vi "Voice coil response and camera trigger_latest.vi"() -> ()   [LabVIEW 2020]
uses:
  <vilib>/DAQmx/read.llb/DAQmx Read (Analog Wfm 1Chan NSamp).vi
  <vilib>/DAQmx/write.llb/DAQmx Write (Analog 1D Wfm NChan NSamp).vi
  <vilib>/DAQmx/create/channels.llb/DAQmx Create Channel (AO-Voltage-Basic).vi
  <vilib>/DAQmx/configure/timing.llb/DAQmx Timing (Use Waveform).vi
  <vilib>/DAQmx/create/channels.llb/DAQmx Create Channel (AI-Voltage-Basic).vi
  <vilib>/DAQmx/configure/timing.llb/DAQmx Timing (Sample Clock).vi
  <vilib>/DAQmx/miscellaneous.llb/DAQmx Fill In Error Info.vi
  <vilib>/Analysis/polynomials.llb/Subtract Polynomials (DBL).vi
  <vilib>/measure/NI_MABase.lvlib
  <vilib>/Analysis/NI_AALPro.lvlib
panel:
  in  "Stop 3":bool
  out "fractional index or x":dbl=9999.0
  out "x/y":dbl=0.5800133152535774
  out "Modified sawtooth input(red) and original sawtooth input (blue)":waveform(dbl)[](graph)=[{"t0"=timestamp(0 s since 1904-01-01), "dt"=0.0001, "Y"=array[10000 elements]}, {"t0"=timestamp(0 s since 1904-01-01), "dt"=0.0001, "Y"=array[10000 elements]}]
  out "intercept":dbl=-0.029693873912173534
  out "slope":dbl=1.09
  out "Linear fit (red), Voice coil response (blue) and Subtracted fit from voice coil response (green)":waveform(dbl)[](graph)=[{"t0"=timestamp(3778592903.950374 s since 1904-01-01), "dt"=9.999999999999999e-05, "Y"=array[10000 elements], "attributes"=variant("NI_ChannelName"=variant(string "Dev1/ai6"), "NI_UnitDescription"=variant(string "Volts"))}, {"t0"=timestamp(0 s since 1904-01-01), "dt"=0.0001, "Y"=array[10000 elements]}, {"t0"=timestamp(0 s since 1904-01-01), "dt"=0.0001, "Y"=array[10000 elements]}]
  in  "Stop 2":bool
  out "Sample Rate":dbl format="%0.2f"
  in  "Camera trigger delay (degrees)":dbl=180.0
  in  "Exposure time (ms)":dbl=1000.0
  in  "Sawtooth Offset":dbl
  in  "Sawtooth Amplitude":dbl=0.2
  in  "Sawtooth Phase":dbl=170.0
  out "Sawtooth input (blue), Voice coil response (red), Voice coil response - Sawtooth input (green)":waveform(dbl)[](graph)=[{"t0"=timestamp(0 s since 1904-01-01), "dt"=0.0001, "Y"=array[10000 elements]}, {"t0"=timestamp(3778592903.950374 s since 1904-01-01), "dt"=9.999999999999999e-05, "Y"=array[10000 elements], "attributes"=variant("NI_ChannelName"=variant(string "Dev1/ai6"), "NI_UnitDescription"=variant(string "Volts"))}, {"t0"=timestamp(0 s since 1904-01-01), "dt"=0.0001, "Y"=array[10000 elements]}]
  out "LabVIEW generated Sawtooth input (blue) and Camera trigger (red)":waveform(dbl)[](graph)=[{"t0"=timestamp(0 s since 1904-01-01), "dt"=0.0001, "Y"=array[10000 elements]}, {"t0"=timestamp(0 s since 1904-01-01), "dt"=0.0001, "Y"=array[10000 elements]}]
  # "Synchronization Settings"
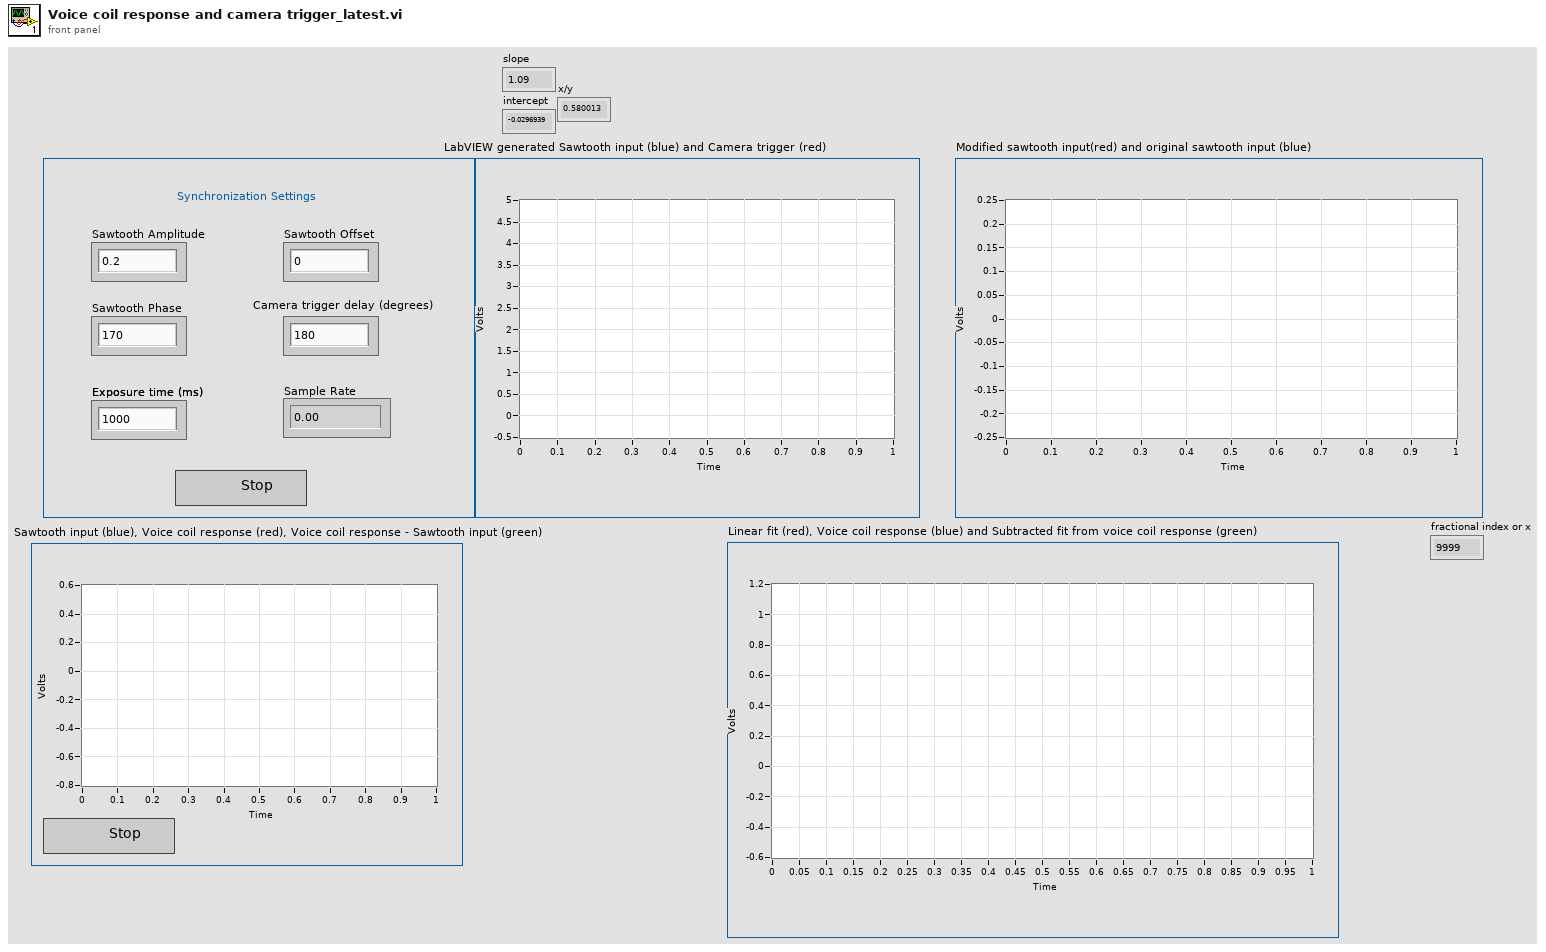
[diagram p1: front panel]
types:
  T1 = cluster{"slope min":dbl, "slope max":dbl, "intercept min":dbl, "intercept max":dbl}
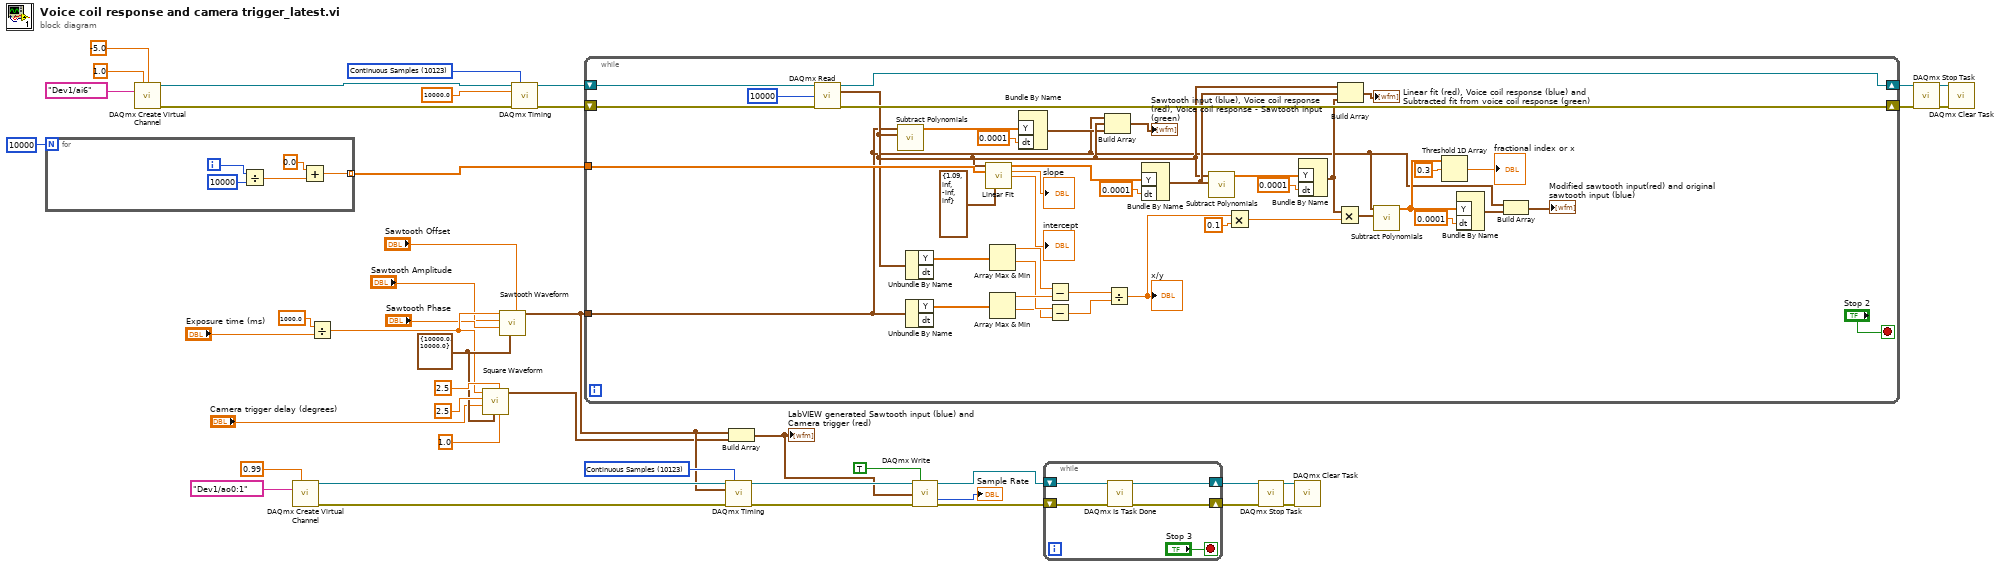
[diagram p0: block diagram]
diagram:
  w31 = 10123 items=["Finite Samples"=10178, "Continuous Samples"=10123, "Hardware Timed Single Point"=12522] ("sample mode")
  w36 = cluster{"Fs":dbl, "#s":dbl} {"Fs"=10000.0, "#s"=10000.0} ("sampling info")
  w41 = 10123 items=["Finite Samples"=10178, "Continuous Samples"=10123, "Hardware Timed Single Point"=12522] ("sample mode")
  n1 = for {
    N: 10000 -> [_]
    tunnel: [w45] -> w16 mode=indexing
    i -> [w49]
    n2 = Divide(x=w49, y=10000) -> (x/y=w46:dbl)
    n3 = Add(x=0.0, y=w46) -> (x+y=w45:dbl)
  }
  n4 = call-poly <vilib>:"DAQmx Create Virtual Channel.vi"("maximum value"=1.0, "minimum value"=-5.0, "physical channels"=tag "Dev1/ai6") -> ("task out"=w34:refnum<k21>, "error out"=w33:errorcluster)  [unwired: 11 in]
  n5 = call-poly <vilib>:"DAQmx Create Virtual Channel.vi"("maximum value"=0.99, "physical channels"=tag "Dev1/ao0:1") -> ("task out"=w43:refnum<k21>, "error out"=w42:errorcluster)  [unwired: 12 in]
  n6 = Divide(x=1000.0, y="Exposure time (ms)") -> (x/y=w35:dbl)
  n7 = call <vilib>:"Square Waveform.vi"("duty cycle (%)"=1.0, "offset"=2.5, "sampling info"=w36, "phase"="Camera trigger delay (degrees)", "amplitude"=2.5, "frequency"=w35) -> ("signal out"=w1:waveform(dbl))  [unwired: 4 in, 1 out]
  n8 = call <vilib>:"Sawtooth Waveform.vi"("offset"="Sawtooth Offset", "sampling info"=w36, "phase"="Sawtooth Phase", "amplitude"="Sawtooth Amplitude", "frequency"=w35) -> ("signal out"=w18:waveform(dbl))  [unwired: 5 in, 1 out]
  n9 = call-poly <vilib>:"DAQmx Timing.vi"("task/channels in"=w34, "sample mode"=w31, "rate"=10000.0, "error in"=w33) -> ("task out"=w30:refnum<k21>, "error out"=w29:errorcluster)  [unwired: 10 in]
  n10 = while {
    shift-right: [w88] -> w26
    shift-left: w30 -> [w90]
    shift-right: [w87] -> w25
    shift-left: w29 -> [w89]
    tunnel: w18 -> [w50]
    tunnel: w16 -> [w81]
    stop <- "Stop 2" stop-if-true
    n11 = call-poly <vilib>:"DAQmx Read.vi"("task/channels in"=w90, "number of samples per channel"=10000, "error in"=w89) -> ("task out"=w88:refnum<k21>, "data"=w69:waveform(dbl), "error out"=w87:errorcluster)  [unwired: 10 in]
    n12 = call-poly <vilib>:"Subtract Polynomials.vi"("Q(x)"=w69, "P(x)"=w50) -> ("P(x)-Q(x)"=w83:dbl[])  [unwired: 8 in, 1 out]
    n13 = Unbundle By Name(w69) -> ("Y"=w68:dbl[])  [unwired: 1 out]
    n14 = Unbundle By Name(w50) -> ("Y"=w67:dbl[])  [unwired: 1 out]
    n15 = call <vilib>:"Linear Fit.vi"("Y"=w69, "X"=w81, "parameter bounds"=T1 {"slope min"=1.09, "slope max"=inf, "intercept min"=-inf, "intercept max"=inf}) -> ("Best Linear Fit"=w79:dbl[], "slope"=→"slope":dbl, "intercept"=→"intercept":dbl)  [unwired: 8 in, 2 out]
    n16 = Array Max & Min(array=w68) -> (max value=w65:dbl, min value=w63:dbl)  [unwired: 2 out]
    n17 = Array Max & Min(array=w67) -> (max value=w66:dbl, min value=w62:dbl)  [unwired: 2 out]
    n18 = Bundle By Name("Y"=w83, "dt"=0.0001) -> (w58:waveform(dbl))  [unwired: 1 in]
    n19 = Subtract(x=w65, y=w66) -> (x-y=w64:dbl)
    n20 = Subtract(x=w63, y=w62) -> (x-y=w61:dbl)
    n21 = Build Array(w50, w69, w58) -> (→"Sawtooth input (blue), Voice coil response (red), Voice coil response - Sawtooth input (green)":waveform(dbl)[])
    n22 = Divide(x=w64, y=w61) -> (x/y=w56:dbl)
    "x/y" <- w56
    n23 = Bundle By Name("Y"=w79, "dt"=0.0001) -> (w77:waveform(dbl))  [unwired: 1 in]
    n24 = call-poly <vilib>:"Subtract Polynomials.vi"("Q(x)"=w77, "P(x)"=w69) -> ("P(x)-Q(x)"=w75:dbl[])  [unwired: 8 in, 1 out]
    n25 = Multiply(x=w56, y=0.1) -> (x*y=w59:dbl)
    n26 = Bundle By Name("Y"=w75, "dt"=0.0001) -> (w70:waveform(dbl))  [unwired: 1 in]
    n27 = Multiply(x=w70, y=w59) -> (x*y=w51:waveform(dbl))
    n28 = Build Array(w69, w77, w70) -> (→"Linear fit (red), Voice coil response (blue) and Subtracted fit from voice coil response (green)":waveform(dbl)[])
    n29 = call-poly <vilib>:"Subtract Polynomials.vi"("Q(x)"=w51, "P(x)"=w50) -> ("P(x)-Q(x)"=w53:dbl[])  [unwired: 8 in, 1 out]
    n30 = Threshold 1D Array(2:0.3 ("threshold y"), 3:w53) -> (0:→"fractional index or x":dbl)  [unwired: 1 in]
    n31 = Bundle By Name("Y"=w53, "dt"=0.0001) -> (w55:waveform(dbl))  [unwired: 1 in]
    n32 = Build Array(w50, w55) -> (→"Modified sawtooth input(red) and original sawtooth input (blue)":waveform(dbl)[])
  }
  n33 = call-poly <vilib>:"DAQmx Timing.vi"("task/channels in"=w43, "sample mode"=w41, "waveform"=w18, "error in"=w42) -> ("task out"=w9:refnum<k21>, "error out"=w7:errorcluster)  [unwired: 10 in]
  n34 = Build Array(w18, w1) -> (w2:waveform(dbl)[])
  "LabVIEW generated Sawtooth input (blue) and Camera trigger (red)" <- w2
  n35 = call-poly <vilib>:"DAQmx Write.vi"("task/channels in"=w9, "auto start"=TRUE, "data"=w2, "error in"=w7) -> ("task out"=w4:refnum<k21>, "number of samples written per channel"=→"Sample Rate":u32, "error out"=w3:errorcluster)  [unwired: 9 in]
  n36 = while {
    shift-right: [w92] -> w6
    shift-left: w4 -> [w95]
    shift-right: [w93] -> w5
    shift-left: w3 -> [w94]
    stop <- "Stop 3" stop-if-true
    n37 = call <vilib>:"DAQmx Is Task Done.vi"("task/channels in"=w95, "error in"=w94) -> ("task out"=w92:refnum<k21>, "error out"=w93:errorcluster)  [unwired: 11 in, 1 out]
  }
  n38 = call <vilib>:"DAQmx Stop Task.vi"("task/channels in"=w6, "error in"=w5) -> ("task out"=w14:refnum<k21>, "error out"=w15:errorcluster)  [unwired: 12 in]
  n39 = call <vilib>:"DAQmx Clear Task.vi"("task in"=w14, "error in"=w15) -> ()  [unwired: 13 in, 1 out]
  n40 = call <vilib>:"DAQmx Stop Task.vi"("task/channels in"=w26, "error in"=w25) -> ("task out"=w27:refnum<k21>, "error out"=w28:errorcluster)  [unwired: 12 in]
  n41 = call <vilib>:"DAQmx Clear Task.vi"("task in"=w27, "error in"=w28) -> ()  [unwired: 13 in, 1 out]
